vi "Init Events.vi"(8 "error in (no error)":errorcluster, 11 "ElementEditorPanel in":refnum<class "ElementEditorPanel.lvclass">) -> (0 "error out":errorcluster, 3 "ElementEditorPanel out":refnum<class "ElementEditorPanel.lvclass">)   [LabVIEW 2020, in "VolatusGUIControls.lvlib" / "ElementEditorPanel.lvclass"]
uses:
  ElementEditorPanel.lvclass
  ElementEditorPanel.lvclass/ElementEditorPanel.ctl
  Update Control Data.ctl
  Incoming Events.ctl
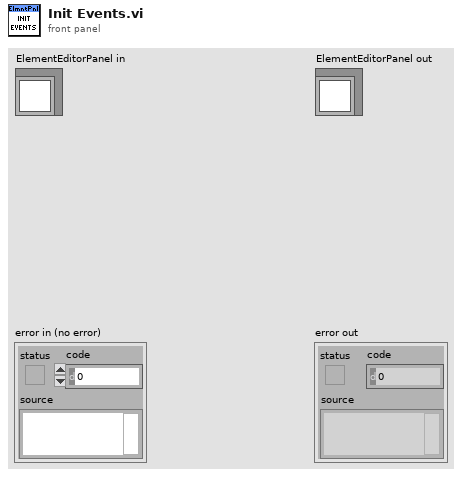
[diagram p1: front panel]
types:
  T1 = typedef "VolatusGUIControls.lvlib/ElementEditorPanel.lvclass/Incoming Events.ctl" = cluster{"Update Control":refnum<user-event>}
  T2 = typedef "VolatusGUIControls.lvlib/ElementEditorPanel.lvclass/Update Control Data.ctl" = cluster{"Ctl Refnum":refnum<vi>}
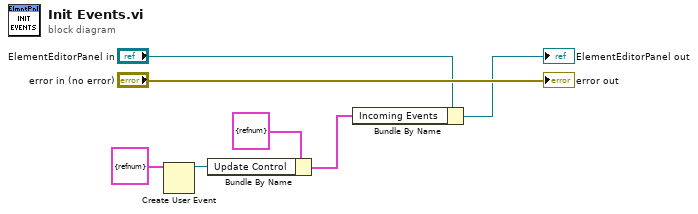
[diagram p0: block diagram]
diagram:
  n1 = Create User Event(user event datatype=T2 {"Ctl Refnum"=refnum} ("Update Control Data")) -> (user event=w3:refnum<user-event>)  [unwired: 1 in, 1 out]
  n2 = Bundle By Name(cluster=T1 {"Update Control"=refnum} ("Incoming Events"), "Update Control"=w3) -> (w1:T1)
  n3 = Bundle By Name(cluster="ElementEditorPanel in", "Incoming Events"=w1) -> (→"ElementEditorPanel out":refnum<class "ElementEditorPanel.lvclass">)
  "error out" <- "error in (no error)"
